vi "MeasureLensThickness.vi"(9 "Compensation factor":dbl, 10 "Refractive index":dbl, 11 "Connection Cluster in":T1) -> (0 "Peak position":dbl, 1 "thickness left":dbl, 2 "thickness right":dbl, 3 "Connection Cluster out":T1)   [LabVIEW 2013]
uses:
  Global.vi
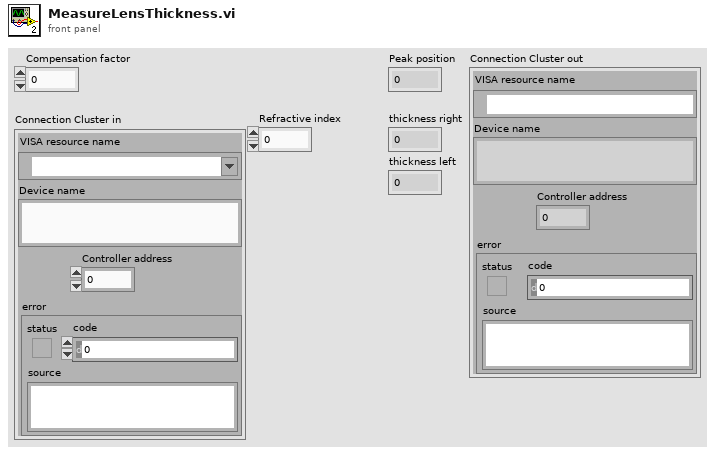
[diagram p1: front panel]
types:
  T1 = cluster{"VISA resource name":refnum<visa-resource-name>, "Device name":string, "Controller address":i32, "error":errorcluster}
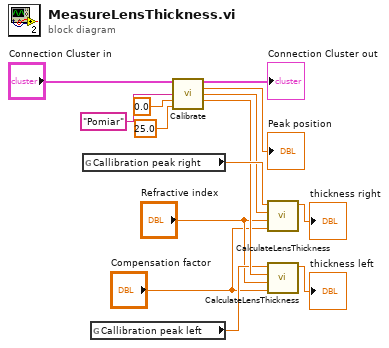
[diagram p0: block diagram]
diagram:
  n1 = global read "Global.vi" "Callibration peak right"() -> (w9:dbl)
  n2 = global read "Global.vi" "Callibration peak left"() -> (w5:dbl)
  n3 = call "Calibrate.vi"("Connection Cluster in"="Connection Cluster in", "String"="Pomiar", "Start position"=0.0, "Target position"=25.0) -> ("Connection Cluster out"=→"Connection Cluster out":T1, "Peak position"=→"Peak position":dbl, "Peak (right)"=w8:dbl, "Peak (left)"=w6:dbl)  [unwired: 8 in]
  n4 = call "CalculateLensThickness.vi"("Compensation factor"="Compensation factor", "Refractive index"="Refractive index", "Measurement Peak Position"=w8, "Callibration Peak Position"=w9) -> ("Lens thickness"=→"thickness right":dbl)  [unwired: 7 in]
  n5 = call "CalculateLensThickness.vi"("Compensation factor"="Compensation factor", "Refractive index"="Refractive index", "Measurement Peak Position"=w6, "Callibration Peak Position"=w5) -> ("Lens thickness"=→"thickness left":dbl)  [unwired: 7 in]
